vi "Accelerometer.vi"(0 "data":string) -> (1 "accel_Y":dbl, 2 "accel_Z":dbl, 3 "accel_X":dbl)   [LabVIEW 2014]
doc: "Extracts the acceleration information from the sensor data"
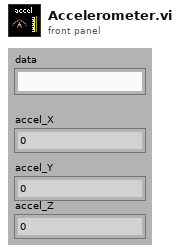
[diagram p1: front panel]
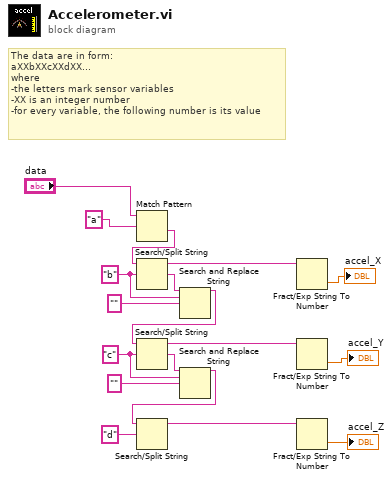
[diagram p0: block diagram]
diagram:
  w14 = "c" ("search string/char (-)")
  w17 = "b" ("search string/char (-)")
  # "The data are in form:\naXXbXXcXXdXX...\nwhere \n-the letters mark sensor variables\n-XX is an integer number\n-for every variable, the following number is its value"
  n1 = Match Pattern(string="data", regular expression="a" ("search string/char (-)")) -> (after substring=w4:string)  [unwired: 1 in, 3 out]
  n2 = Search/Split String(string=w4, search string/char (-)=w17) -> (substring before match=w8:string, match + rest of string=w18:string)  [unwired: 1 in, 1 out]
  n3 = Search and Replace String(input string=w18, search string=w17, replace string="" ("replace string (\"\")")) -> (result string=w12:string)  [unwired: 5 in, 3 out]
  n4 = Search/Split String(string=w12, search string/char (-)=w14) -> (substring before match=w7:string, match + rest of string=w13:string)  [unwired: 1 in, 1 out]
  n5 = Search and Replace String(input string=w13, search string=w14, replace string="" ("replace string (\"\")")) -> (result string=w10:string)  [unwired: 5 in, 3 out]
  n6 = Search/Split String(string=w10, search string/char (-)="d") -> (substring before match=w6:string)  [unwired: 1 in, 2 out]
  n7 = Fract/Exp String To Number(string=w8) -> (number=→"accel_X":dbl)  [unwired: 3 in, 1 out]
  n8 = Fract/Exp String To Number(string=w7) -> (number=→"accel_Y":dbl)  [unwired: 3 in, 1 out]
  n9 = Fract/Exp String To Number(string=w6) -> (number=→"accel_Z":dbl)  [unwired: 3 in, 1 out]
